vi "MAIN_GLD.vi"() -> ()   [LabVIEW 2019]
uses:
  <vilib>/platform/TimedLoop/XDataNode/XDataNode.xnode
  <vilib>/Platform/TimedLoop/XDataNode/nitl_modes.ctl
  <vilib>/Platform/TimedLoop/XDataNode/XDNodeRunTimeDep.lvlib
  <vilib>/Platform/TimedLoop/XDataNode/wakeup.ctl
  <vilib>/Platform/TimedLoop/XDataNode/timing_clust.ctl
  For fsr type def.ctl
  states typedef.ctl
  <vilib>/Analysis/NI_AALBase.lvlib
  <vilib>/Analysis/baseanly.llb/Mean (DBL).vi
  TESTtypedef UPDATED.ctl
  <extravilib>/ChannelInstances/Tag-bool.lvlib
  SineMinMax.ctl
  <vilib>/Instr/_visa.llb/VISA Configure Serial Port (Instr).vi
  weightTypedef.ctl
  groupID.ctl
  handInTest.ctl
  RampSlope.ctl
  RampHeight.ctl
panel:
  out "LF":dbl(graph)
  out "GF":dbl(graph)
  in  "Ramp's Height (N)":T1
  in  "Sine Min/Max (N)":T2=5.0
  out "Writing":bool
  in  "Stop Test":bool
  out "Grip Force [N]":cluster{"GF [N]":dbl}(graph)
  out "XY Graph":cluster{dbl[], dbl[]}[](graph)
  out "Test Time":dbl(graph)
  in  "Ramp's Width (s)":T3 caption="Test Type"
  in  "VISA":refnum<visa-resource-name>="COM1"
  out "Load Force [N]":cluster{"Dyna LF [N]":dbl}(graph)
  out "In Range?":bool
  in  "Wait time before beep (s)":dbl
  in  "Time b/w Beeps (s)":dbl=3.0
  in  "Stop":bool
  out "?":string
  in  "File Path":path=path "C:/Users/rsKite/Documents/Data_logs"
  out "Creating":bool
  in  "Create File":bool
  in  "Wrist Angle":enum16{"0", "30", "-30"}(ring)
  in  "Hand in Test":T4 caption="Test Type"
  in  "Trial":string caption="Participant Name (FirstLast)"
  in  "Patient ID":string caption="Participant Name (FirstLast)"
  in  "Group ID":T5
  in  "Weight":T6
  in  "Test Type":T7
  in  "Start Test":bool
  out "Calibrating":bool
  in  "Calibration":bool
  in  "Timer [ms]":u32=5000
  out "millisecond timer":u32
  out "dt":dbl
  out "millisecond timer 2":u32
  # "Status"
  # "Grip-Load Hand Assessment Device  Control Center"
  # "Control"
  # "Test Setup"
  # "File Control"
  # "Folder/File Information"
  # "STUFF THAT DOES NOT NEED TO BE DISPLAYED"
  # "Test Control"
  # "Force/Motion Trajectory Control"
  # "Test Time (s)"
  # "Grip Force"
  # "Load Force"
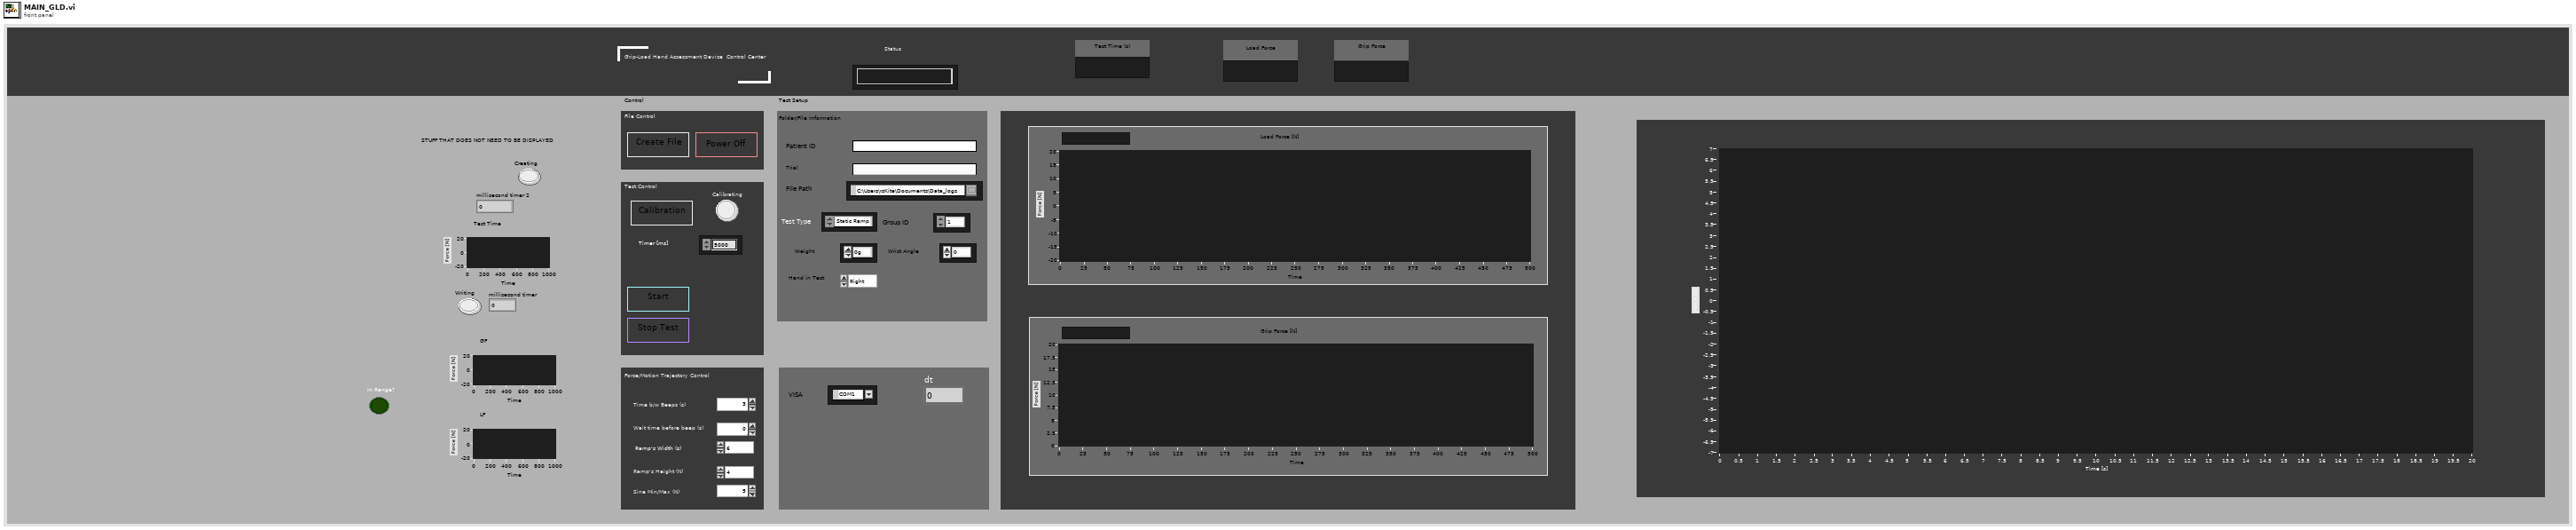
[diagram p1: front panel]
types:
  T1 = typedef "RampHeight.ctl" = enum16{"4", "5", "6"}
  T2 = typedef "SineMinMax.ctl" = dbl
  T3 = typedef "RampSlope.ctl" = enum16{"6", "5", "4"}
  T4 = typedef "handInTest.ctl" = enum16{"Right", "Left"}
  T5 = typedef "groupID.ctl" = enum16{"1", "2"}
  T6 = typedef "weightTypedef.ctl" = enum16{"0g", "300g", "600g", "900g"}
  T7 = typedef "TESTtypedef UPDATED.ctl" = enum16{"Static Ramp", "Static Sine", "Dynamic"}
  T8 = cluster{"String 2":string, dbl[], dbl[], dbl[], dbl[], dbl[], dbl[], dbl[], dbl[], "Test Type":T7, "Sine Min/Max (N) ":T2, "Ramp's Width":dbl, "Ramp's Height":dbl, dbl, dbl[]}
  T9 = typedef "states typedef.ctl" = enum16{"Init", "Create/Replace", "Calibration", "Ready?", "Testing", "Write Data", "Restart"}
  T10 = typedef "For fsr type def.ctl" = enum16{"Create/Replace File", "Waiting Room", "Collect Data", "Write Data", "Close File", "Reinit"}
  T11 = typedef "XDNodeRunTimeDep.lvlib/timing_clust.ctl" = cluster{"Expected End [f-1]":u64, "Actual End [f-1]":u64, "Finished Late? [f-1]":bool, "Expected End [i-1]":u64, "Actual End [i-1]":u64, "Finished Late? [i-1]":bool, "Expected Start [i]":u64, "Actual Start [i]":u64, "Expected Start [f]":u64, "Actual Start [f]":u64, "Source Name":string, "Structure Name":string, "Period":i64, "Deadline":i64, "Offset":i64, "Start":i64, "Priority":i32, "Timeout":i32, "Mode":T12, "Wakeup Reason":T13, "Error":errorcluster, "Source Type":string, "Secondary Source Type":string, "Global End Time":u64, "Global Start Time":u64, "Frame Duration":u64, "Iteration Duration":u64, "Assigned CPU":i32, "I/O Scan Engine Mode":u32}
  T12 = typedef "XDNodeRunTimeDep.lvlib/nitl_modes.ctl" = enum32{"No Change", "Process missed periods, maintain original phase", "Discard missed periods, maintain original phase", "Process missed periods, ignore original phase", "Discard missed periods, ignore original phase"}
  T13 = typedef "XDNodeRunTimeDep.lvlib/wakeup.ctl" = enum32{"Normal", "Aborted", "Asynchronous wakeup", "Timing source error", "Timed loop error", "Timeout"}
  T14 = cluster{"Foldername and filename string":string, dbl[], dbl[], dbl[], dbl[], "output array":dbl[], "output array":dbl[], "output array":dbl[], "output array":dbl[], "Test Type":T7, "Sine Min/Max (N) ":T2, "Ramp's Width":dbl, "Ramp's Height":dbl, dbl, "output array":dbl[]}
  T15 = cluster{"String 2":string, dbl[], dbl[], dbl[], dbl[], "array":dbl[], dbl[], dbl[], "output array":dbl[], "Test Type":T7, "Sine Min/Max (N) ":T2, "Ramp's Width":dbl, "Ramp's Height":dbl, dbl, dbl[]}
  T16 = cluster{"String 2":string, dbl[], dbl[], dbl[], dbl[], "array":dbl[], "output array":dbl[], "output array":dbl[], dbl[], "Test Type":T7, "Sine Min/Max (N) ":T2, "Ramp's Width":dbl, "Ramp's Height":dbl, dbl, "output array":dbl[]}
  T17 = typedef "Tag-bool.lvlib/))Channel.ctl" = refnum<queue>
  T18 = cluster{"refnum out":refnum<file>, "error out":errorcluster}
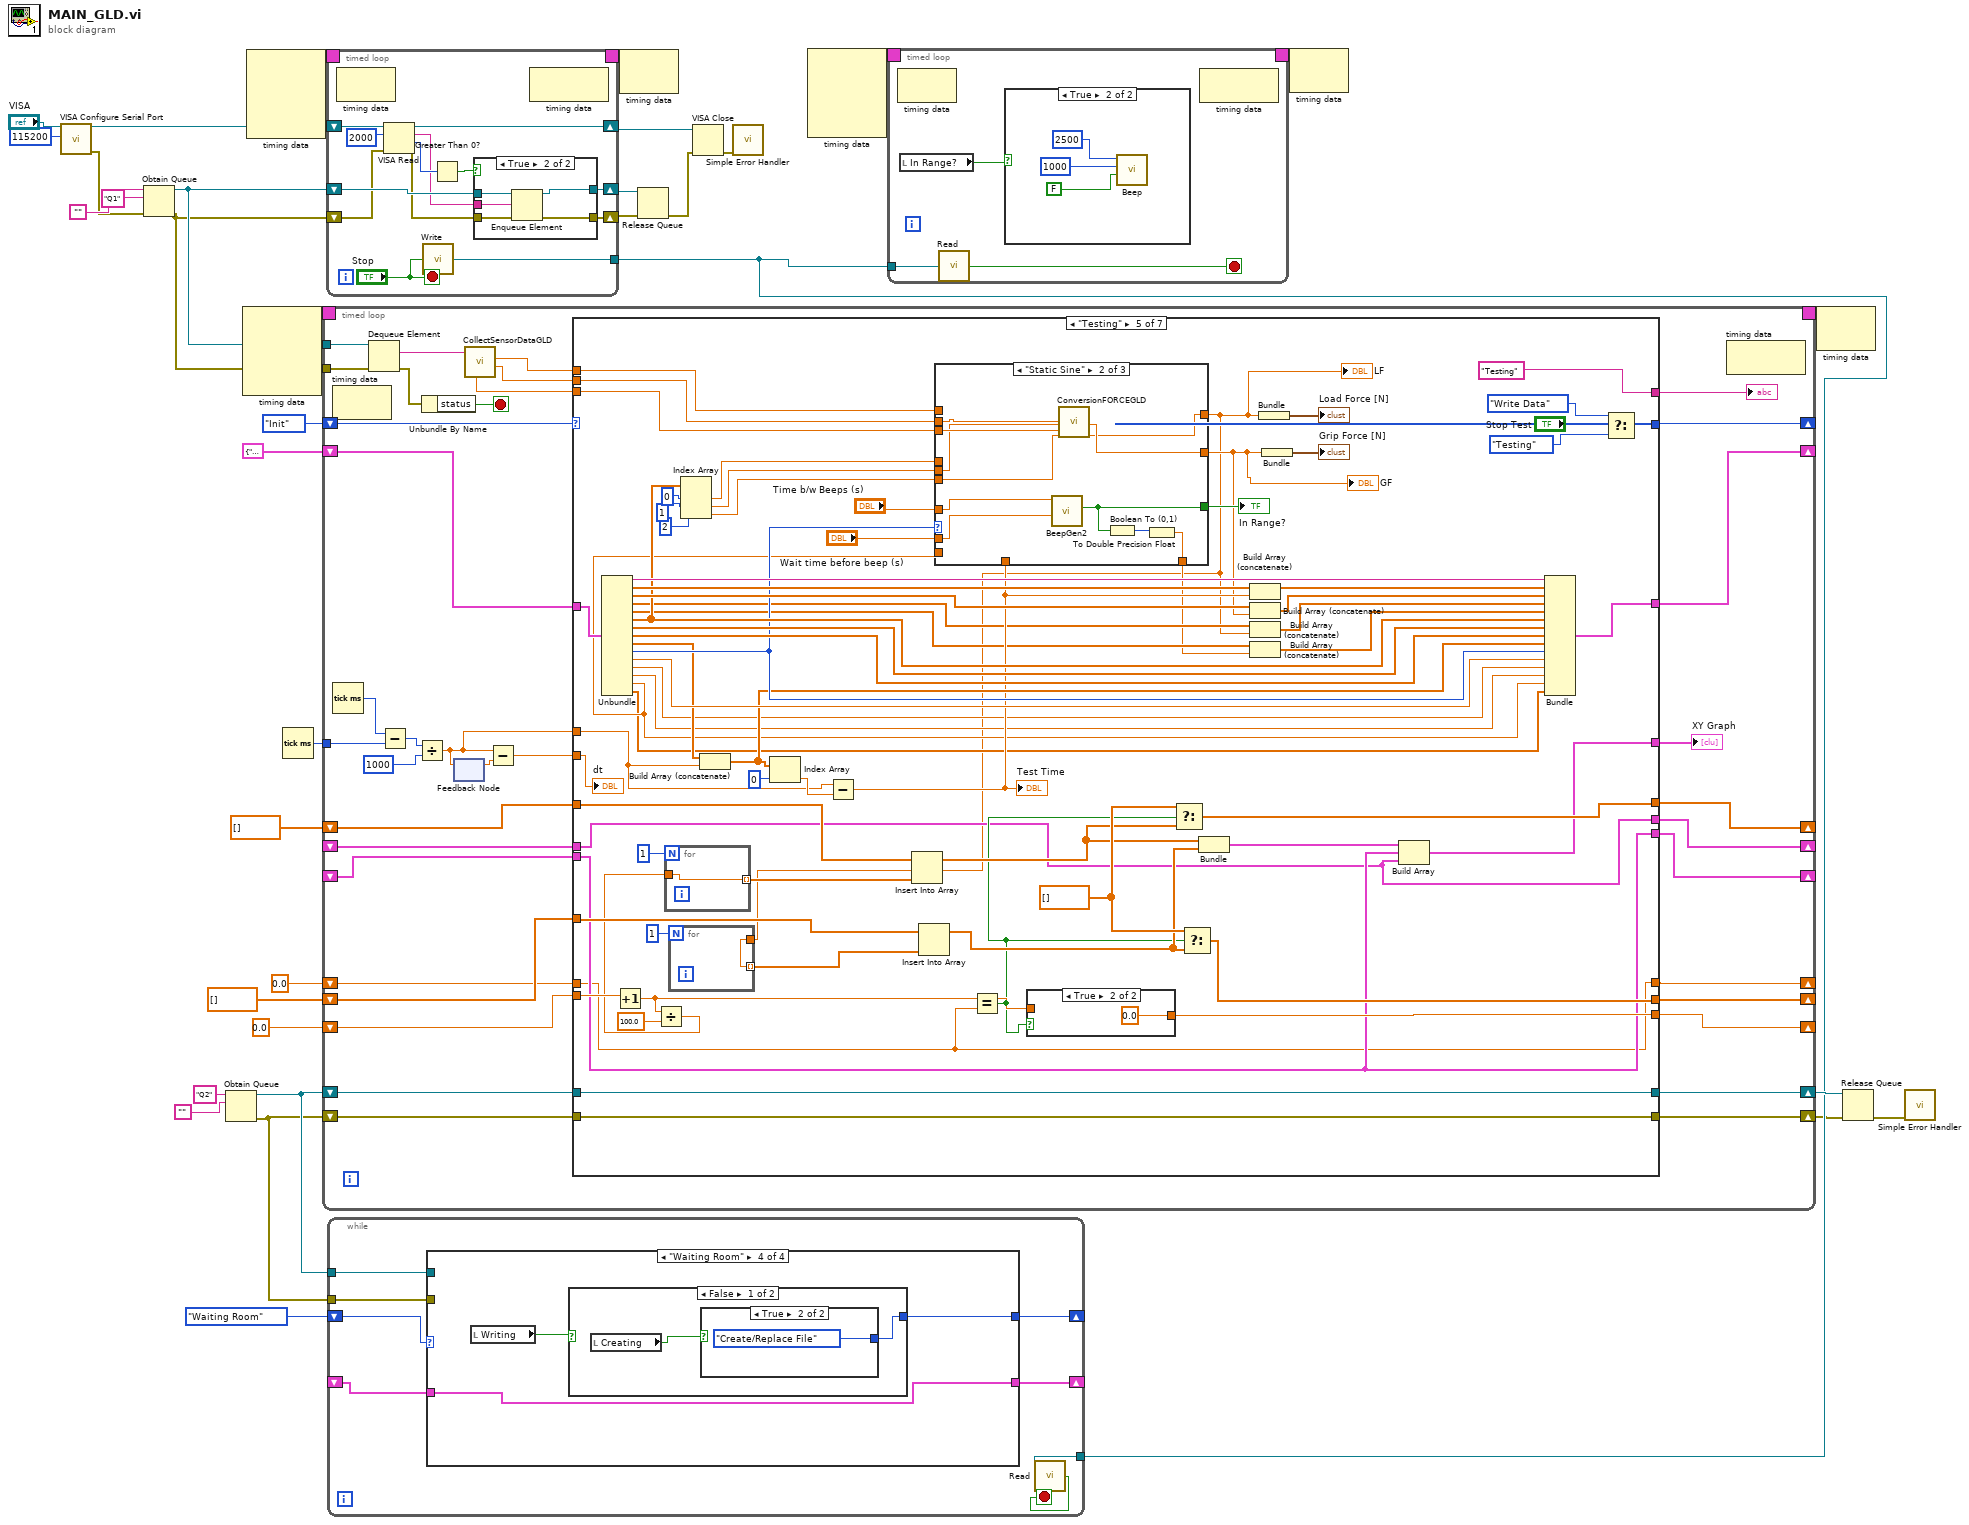
[diagram p0: block diagram]
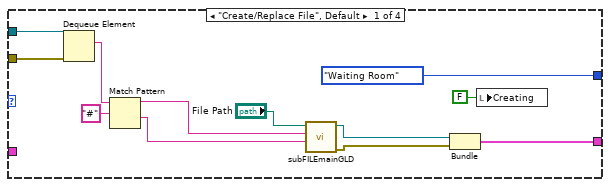
[diagram p3: hidden frame]
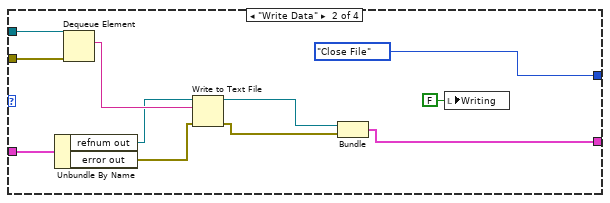
[diagram p4: hidden frame]
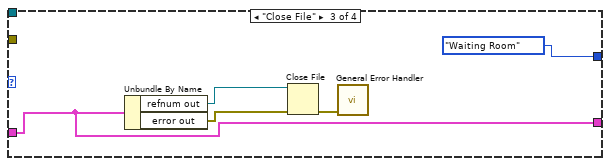
[diagram p5: hidden frame]
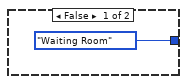
[diagram p6: hidden frame]
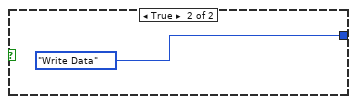
[diagram p7: hidden frame]
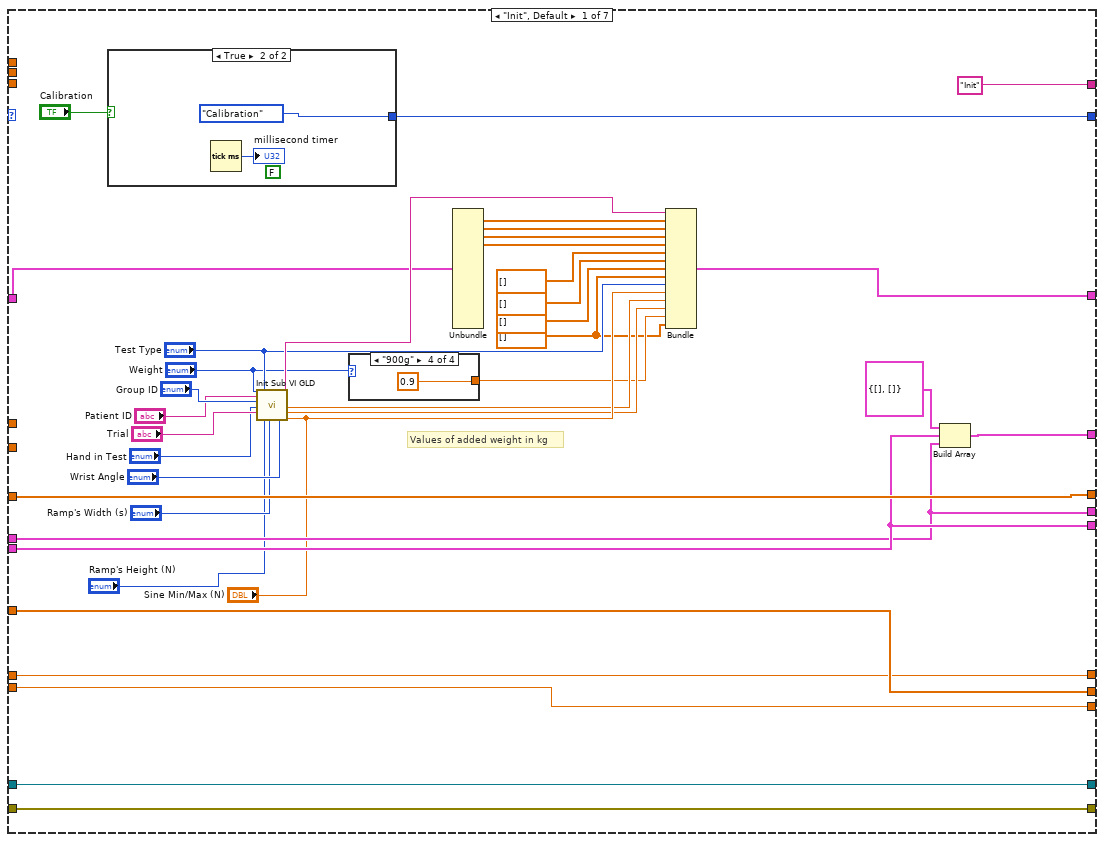
[diagram p8: hidden frame]
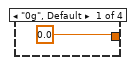
[diagram p9: hidden frame]
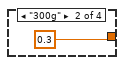
[diagram p10: hidden frame]
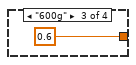
[diagram p11: hidden frame]
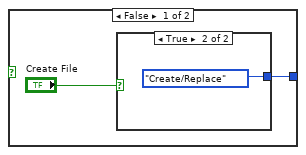
[diagram p12: hidden frame]
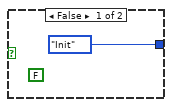
[diagram p13: hidden frame]
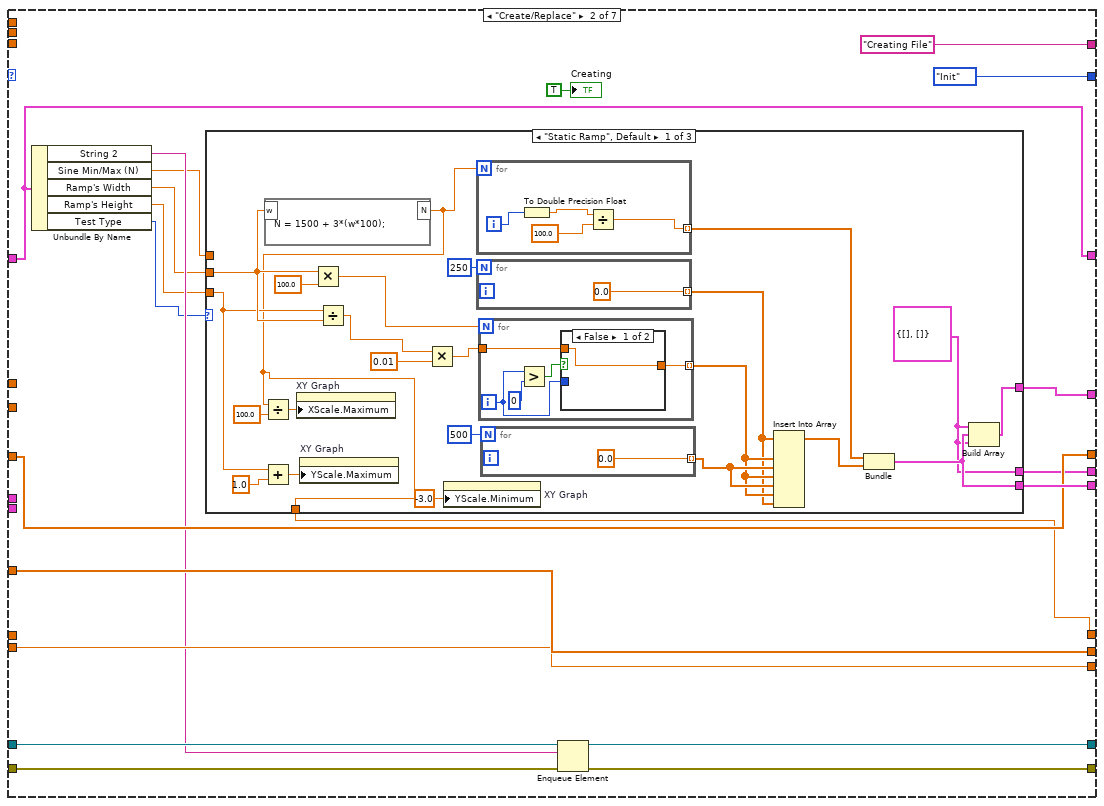
[diagram p14: hidden frame]
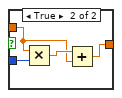
[diagram p15: hidden frame]
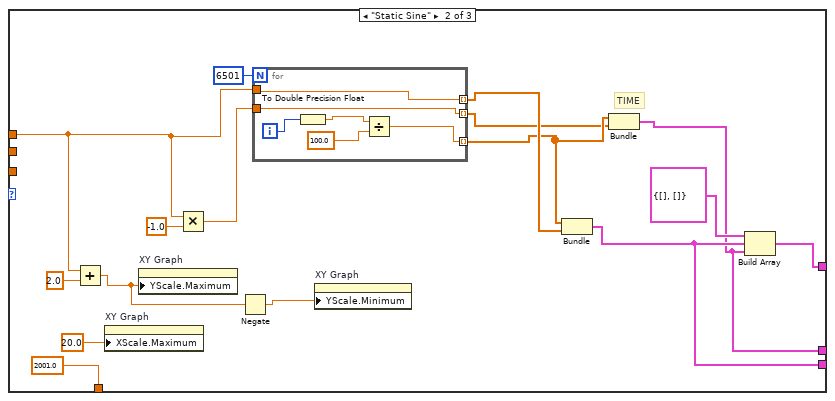
[diagram p16: hidden frame]
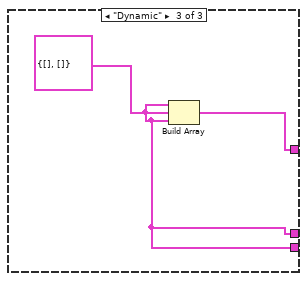
[diagram p17: hidden frame]
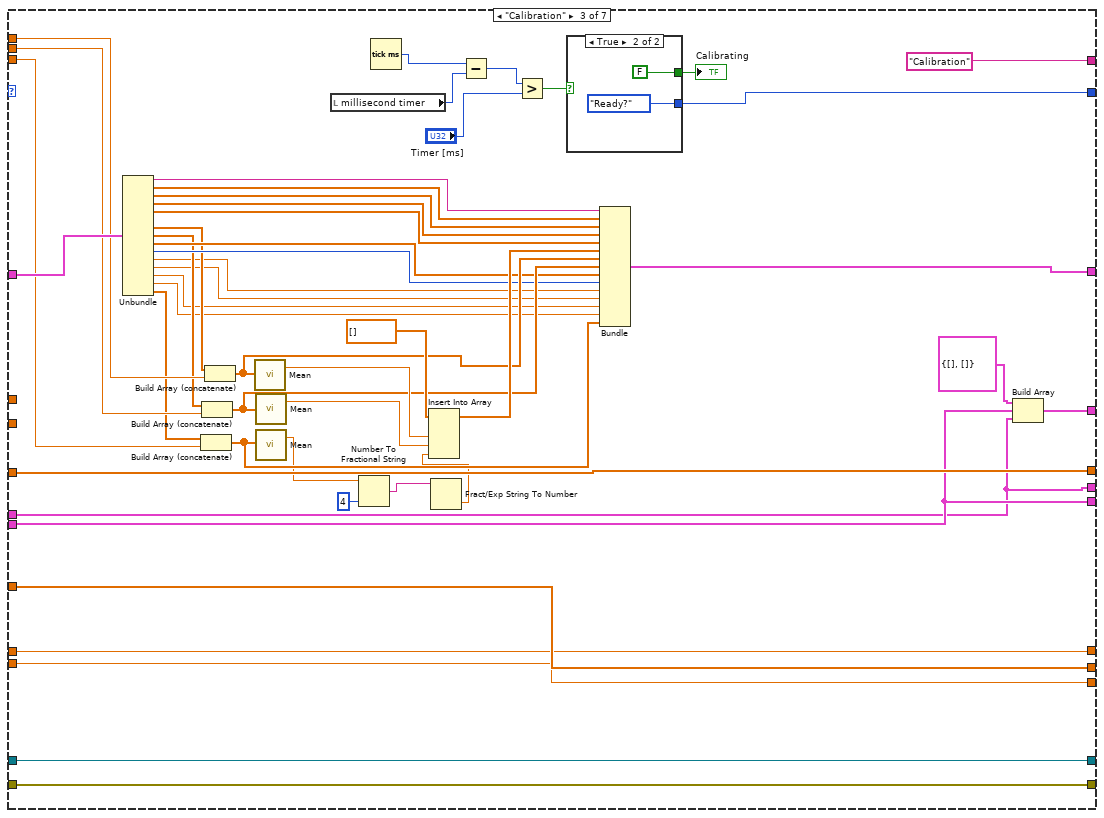
[diagram p18: hidden frame]
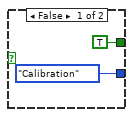
[diagram p19: hidden frame]
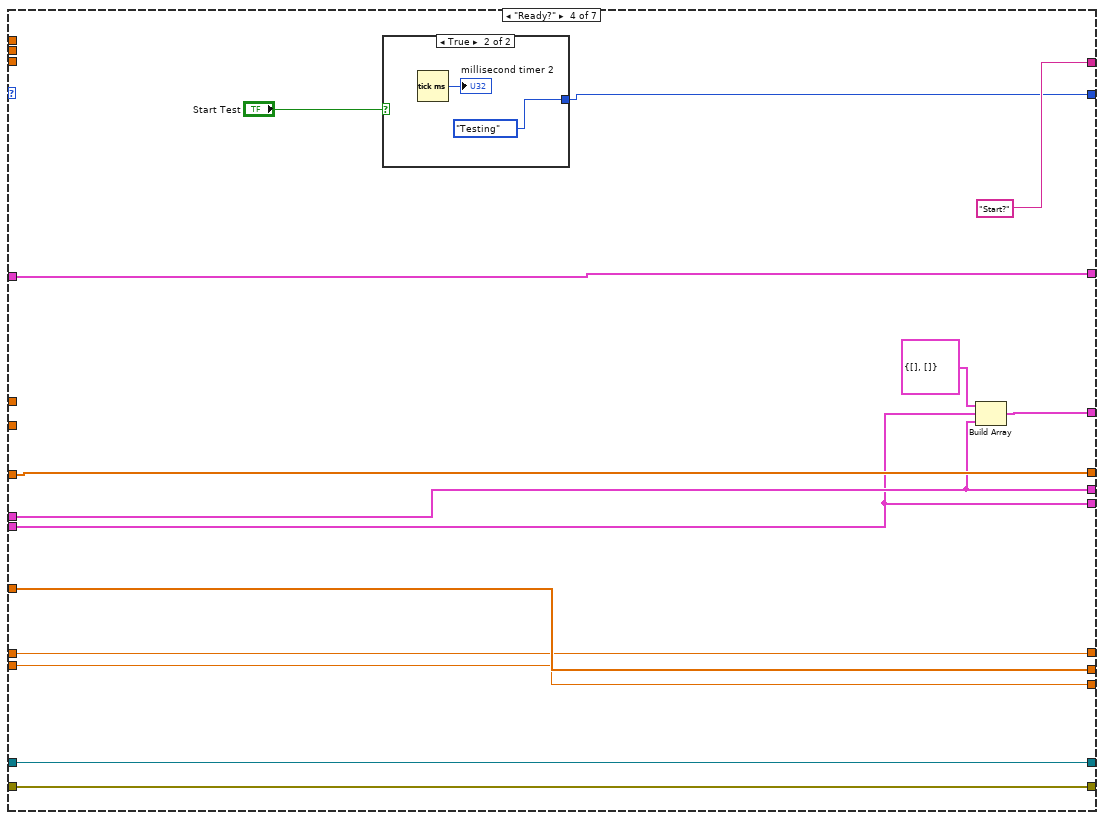
[diagram p20: hidden frame]
diagram:
  n1 = call-poly "VISA Configure Serial Port"("VISA resource name"="VISA", "baud rate (9600)"=u32 115200) -> ("VISA resource name out"=w31:refnum<visa-resource-name>, "error out"=w26:errorcluster)  [unwired: 12 in]
  n2 = Obtain Queue(name (unnamed)="Q1", element data type="", error in (no error)=w26) -> (queue out=w33:refnum<queue>, error out=w32:errorcluster)  [unwired: 2 in, 1 out]
  n3 = Obtain Queue(name (unnamed)="Q2", element data type="") -> (queue out=w17:refnum<queue>, error out=w16:errorcluster)  [unwired: 3 in, 1 out]
  n4 = node-c288() -> (w21:T11)  [unwired: 4 in]
  n5 = node-c288() -> (w23:T11)  [unwired: 4 in]
  n6 = Tick Count (ms)() -> (millisecond timer value=w24:u32)
  n7 = timed-loop {
    tunnel: w33 -> [w72]
    tunnel: w32 -> [w71]
    tunnel: w24 -> [w68]
    timing: w21 -> [_]
    timing-out: [_] -> w20
    shift-right: [w60] -> _
    shift-left: states_typedef."Init" -> [w59]
    shift-right: [w62] -> w15
    shift-left: w17 -> [w64]
    shift-right: [w61] -> w2
    shift-left: w16 -> [w63]
    shift-right: [w56] -> _
    shift-left: T8 {"String 2"="", [], [], [], [], [], [], [], [], "Test Type"=enum."Dynamic", "Sine Min/Max (N) "=3000.0, "Ramp's Width"=0.0, "Ramp's Height"=0.0, 0.0, []} -> [w57]
    shift-right: [w53] -> _
    shift-left: _ -> [w52]
    shift-right: [w45] -> _
    shift-left: dbl[] [] ("t") -> [w46]
    shift-right: [w44] -> _
    shift-left: dbl[] [] ("t") -> [w43]
    shift-right: [w40] -> _
    shift-left: 0.0 -> [w41]
    shift-right: [w39] -> _
    shift-left: _ -> [w38]
    shift-right: [w37] -> _
    shift-left: 0.0 ("Y Scale.Range:Maximum") -> [w36]
    stop <- w55 stop-if-true
    n8 = node-c288() -> ()  [unwired: 1 in, 1 out]
    n9 = Tick Count (ms)() -> (millisecond timer value=w69:u32)
    n10 = Dequeue Element(queue=w72, error in (no error)=w71) -> (element=w58:string, error out=w70:errorcluster)  [unwired: 1 in, 2 out]
    n11 = Subtract(x=w69, y=w68) -> (x-y=w66:u32)
    n12 = Divide(x=w66, y=1000) -> (x/y=w51:dbl)
    n13 = Unbundle By Name(w70) -> ("status"=w55:bool)
    n14 = feedback-in #1(w51) -> ()
    n15 = feedback #1() -> (w65:dbl)  [unwired: 1 in]
    n16 = call "CollectSensorDataGLD.vi"("data (can be any type)"=w58) -> ("grams (GF)"=w47:dbl, "Accel (Dyna LF)"=w48:dbl, "Volt (Static LF)"=w49:dbl)  [unwired: 8 in]
    n17 = Subtract(x=w51, y=w65) -> (x-y=w50:dbl)
    n18 = case shown="\"Testing\"" w59 {
      tunnel: [w109 states_typedef."Init" w241 w263 w313 states_typedef."Restart" states_typedef."Init"] -> w60
      tunnel: w64 -> [w107 w139 w240 w267 w344 w409 w426]
      tunnel: w63 -> [w106 w121 w239 w266 w343 w408 w425]
      tunnel: [w107 w138 w240 w267 w344 w407 w426] -> w62
      tunnel: [w106 w137 w239 w266 w343 w406 w425] -> w61
      tunnel: w57 -> [w90 w127 w238 w265 w340 w404 _]
      tunnel: [w95 w127 w231 w265 w335 w404 T8 {"String 2"="", [], [], [], [], [], [], [], [], "Test Type"=enum."Dynamic", "Sine Min/Max (N) "=3000.0, "Ramp's Width"=0.0, "Ramp's Height"=0.0, 0.0, []}] -> w56
      tunnel: ["Init" "Creating File" "Calibration" "Start?" "Testing" "Logging" "Restarting"] -> w54
      tunnel: [w86 w133 w217 w256 w290 w396 w420] -> w53
      tunnel: w52 -> [w86 _ w217 w256 w290 w396 w420]
      tunnel: w51 -> [_ _ _ _ w331 _ _]
      tunnel: w48 -> [_ _ w229 _ w330 _ _]
      tunnel: w50 -> [_ _ _ _ w329 _ _]
      tunnel: w49 -> [_ _ w210 _ w325 _ _]
      tunnel: w47 -> [_ _ w211 _ w326 _ _]
      tunnel: w46 -> [w88 w132 w221 w261 w307 w399 _]
      tunnel: [w88 w132 w221 w261 w309 w399 dbl[] [] ("t")] -> w45
      tunnel: [w87 w131 w220 w262 w308 w398 dbl[] [] ("t")] -> w44
      tunnel: w43 -> [w87 w131 w220 w262 w304 w398 _]
      tunnel: [w85 w130 w213 w260 w298 w397 w419] -> w42
      tunnel: w41 -> [w84 w129 w219 w259 w297 w395 _]
      tunnel: [w84 w129 w219 w259 w296 w395 0.0] -> w40
      tunnel: [w81 w128 w216 w257 w289 w393 w416] -> w39
      tunnel: w38 -> [w81 _ w216 w257 w289 w393 w416]
      tunnel: [w73 w120 w203 w255 w274 w383 0.0 ("Y Scale.Range:Maximum")] -> w37
      tunnel: w36 -> [w73 _ w203 w255 w274 w383 _]
      frame "Init", Default {
        w74 = dbl[] [] ("output array")
        # "Values of added weight in kg"
        n19 = case shown="True" "Calibration" {
          tunnel: [w115 states_typedef."Calibration"] -> w109
          frame False {
            n20 = case shown="True" "Create File" {
              tunnel: [states_typedef."Init" states_typedef."Create/Replace"] -> w115
              frame False {
                (unwired) FALSE
              }
              frame True {
              }
            }
          }
          frame True {
            (unwired) FALSE
            n21 = Tick Count (ms)() -> (millisecond timer value=→"millisecond timer":u32)
          }
        }
        n22 = call "Init Sub VI GLD.vi"("Weight"="Weight", "Patient ID"="Patient ID", "Group ID"="Group ID", "Hand in Test"="Hand in Test", "Trial"="Trial", "Test Type"="Test Type", "Ramp's Height (N)"="Ramp's Height (N)", "Ramp's Width (s)"="Ramp's Width (s)", "Wrist Angle"="Wrist Angle", "Sine Min/Max"="Sine Min/Max (N)") -> ("Foldername and filename string"=w94:string, "Ramp's Width"=w78:dbl, "Ramp's Height"=w77:dbl)  [unwired: 6 in, 1 out]
        n23 = case shown="\"900g\"" "Weight" {
          tunnel: [0.0 0.3 0.6 0.9] -> w75
          frame "0g", Default {
          }
          frame "300g" {
          }
          frame "600g" {
          }
          frame "900g" {
          }
        }
        n24 = Unbundle(w90) -> (w100:dbl[], w99:dbl[], w98:dbl[], w97:dbl[])  [unwired: 11 out]
        n25 = Bundle("Foldername and filename string"=w94, w100, w99, w98, w97, "output array"=dbl[] [], "output array"=dbl[] [], "output array"=dbl[] [], "output array"=w74, "Test Type"="Test Type", "Sine Min/Max (N)"="Sine Min/Max (N)", "Ramp's Width"=w78, "Ramp's Height"=w77, w75, "output array"=w74) -> (w95:T14)  [unwired: 1 in]
        n26 = Build Array(cluster{dbl[], dbl[]} {[], []} ("element"), w86, w81) -> (w85:cluster{dbl[], T2[]}[])
      }
      frame "Create/Replace" {
        n27 = Unbundle By Name(w127) -> ("String 2"=w126:string, "Sine Min/Max (N)"=w124:T2, "Ramp's Width"=w123:dbl, "Ramp's Height"=w122:dbl, "Test Type"=w125:T7)
        n28 = case shown="\"Static Ramp\", Default" w125 {
          tunnel: [w161 w193 w201] -> w133
          tunnel: w123 -> [w147 _ _]
          tunnel: [w159 w194 w202] -> w130
          tunnel: w124 -> [_ w183 _]
          tunnel: [w158 w187 w201] -> w128
          tunnel: w122 -> [w145 _ _]
          tunnel: [w141 2001.0 ("Y Scale.Range:Maximum") _] -> w120
          frame "Static Ramp", Default {
            w158 = cluster{dbl[], dbl[]} {[], []} ("element")
            n29 = Add(x=w145, y=1.0) -> (x+y=w143:dbl)
            n30 = formula code="N = 1500 + 3*(w*100);"("w"=w147) -> ("N"=w141:dbl)
            n31 = Divide(x=w141, y=100.0) -> (x/y=w142:dbl)
            n32 = property on="XY Graph" class="XYGraph (strict)"("XScale.Maximum"=w142) -> ()  [unwired: 2 in, 2 out]
            n33 = property on="XY Graph" class="XYGraph (strict)"("YScale.Maximum"=w143) -> ()  [unwired: 2 in, 2 out]
            n34 = Multiply(x=w147, y=100.0) -> (x*y=w155:dbl)
            n35 = Divide(x=w145, y=w147) -> (x/y=w153:dbl)
            n36 = Multiply(x=w153, y=0.01) -> (x*y=w152:dbl)
            n37 = property on="XY Graph" class="XYGraph (strict)"("YScale.Minimum"=-3.0 ("Y Scale.Range:Minimum")) -> ()  [unwired: 2 in, 2 out]
            n38 = for {
              N: w141 -> [_]
              tunnel: [w175] -> w157 mode=indexing
              i -> [w178]
              n39 = To Double Precision Float(number=w178) -> (double precision float=w176:dbl)
              n40 = Divide(x=w176, y=100.0) -> (x/y=w175:dbl)
            }
            n41 = for {
              N: 250 -> [_]
              tunnel: [0.0] -> w148 mode=indexing
            }
            n42 = for {
              N: w155 -> [_]
              tunnel: w152 -> [w166]
              tunnel: [w165] -> w149 mode=indexing
              i -> [w164]
              n43 = Greater?(x=w164, y=0) -> (0:w167:bool)
              n44 = case shown="False" w167 {
                tunnel: w166 -> [w169 w171]
                tunnel: [w169 w170] -> w165
                tunnel: w164 -> [_ w173]
                frame False {
                }
                frame True {
                  n45 = Multiply(x=w171, y=w173) -> (x*y=w172:dbl)
                  n46 = Add(x=w172, y=w171) -> (x+y=w170:dbl)
                }
              }
            }
            n47 = for {
              N: 500 -> [_]
              tunnel: [0.0] -> w150 mode=indexing
            }
            n48 = Insert Into Array(array=w148, new element #1=w149, new element #2=w150, new element #3=w149, new element #4=w150, new element #5=w149, new element #6=w148) -> (w162:dbl[])  [unwired: 1 in]
            n49 = Bundle(w157, w162) -> (w161:cluster{dbl[], dbl[]})  [unwired: 1 in]
            n50 = Build Array(w158, w161, w158) -> (w159:cluster{dbl[], dbl[]}[])
          }
          frame "Static Sine" {
            # "TIME"
            n51 = Add(x=w183, y=2.0) -> (x+y=w181:T2)
            n52 = property on="XY Graph" class="XYGraph (strict)"("XScale.Maximum"=20.0 ("Y Scale.Range:Maximum")) -> ()  [unwired: 2 in, 2 out]
            n53 = property on="XY Graph" class="XYGraph (strict)"("YScale.Maximum"=w181) -> ()  [unwired: 2 in, 2 out]
            n54 = Multiply(x=w183, y=-1.0) -> (x*y=w185:T2)
            n55 = Negate(x=w181) -> (-x=w180:T2)
            n56 = for {
              N: 6501 -> [_]
              tunnel: [w196] -> w192 mode=indexing
              tunnel: [w197] -> w191 mode=indexing
              tunnel: w183 -> [w196]
              tunnel: w185 -> [w195]
              tunnel: [w195] -> w186 mode=indexing
              i -> [w200]
              n57 = To Double Precision Float(number=w200) -> (double precision float=w198:dbl)
              n58 = Divide(x=w198, y=100.0) -> (x/y=w197:dbl)
            }
            n59 = property on="XY Graph" class="XYGraph (strict)"("YScale.Minimum"=w180) -> ()  [unwired: 2 in, 2 out]
            n60 = Bundle(w191, w192) -> (w193:cluster{dbl[], T2[]})  [unwired: 1 in]
            n61 = Bundle(w191, w186) -> (w187:cluster{dbl[], T2[]})  [unwired: 1 in]
            n62 = Build Array(cluster{dbl[], T2[]} {[], []} ("element"), w193, w187) -> (w194:cluster{dbl[], T2[]}[])
          }
          frame "Dynamic" {
            w201 = cluster{dbl[], dbl[]} {[], []} ("element")
            n63 = Build Array(w201, w201, w201) -> (w202:cluster{dbl[], dbl[]}[])
          }
        }
        n64 = Enqueue Element(queue=w139, element=w126, error in (no error)=w121) -> (queue out=w138:refnum<queue>, error out=w137:errorcluster)  [unwired: 1 in, 1 out]
        "Creating" <- TRUE ("Creating")
      }
      frame "Calibration" {
        n65 = Unbundle(w238) -> ("String 2"=w237:string, w236:dbl[], w235:dbl[], w234:dbl[], w233:dbl[], "output array"=w224:dbl[], "output array"=w223:dbl[], "output array"=w226:dbl[], "Test Type"=w225:T7, "Sine Min/Max (N)"=w222:T2, "Ramp's Width"=w215:dbl, "Ramp's Height"=w214:dbl, w212:dbl, "output array"=w209:dbl[])  [unwired: 1 out]
        n66 = Build Array (concatenate)(w209, w210) -> (w208:dbl[])
        n67 = Build Array (concatenate)(w223, w211) -> (w227:dbl[])
        n68 = Build Array (concatenate)(w224, w229) -> (w228:dbl[])
        n69 = call-poly <vilib>:"Mean.vi"("X"=w228) -> ("mean"=w249:dbl)  [unwired: 1 out]
        n70 = call-poly <vilib>:"Mean.vi"("X"=w227) -> ("mean"=w248:dbl)  [unwired: 1 out]
        n71 = call-poly <vilib>:"Mean.vi"("X"=w208) -> ("mean"=w206:dbl)  [unwired: 1 out]
        n72 = local read "millisecond timer"() -> (w246:u32)
        n73 = Number To Fractional String(number=w206, precision (6)=i16 4) -> (F-format string=w205:string)  [unwired: 2 in]
        n74 = Tick Count (ms)() -> (millisecond timer value=w247:u32)
        n75 = Fract/Exp String To Number(string=w205) -> (number=w204:dbl)  [unwired: 3 in, 1 out]
        n76 = Insert Into Array(array=dbl[] [], new element #1=w249, new element #2=w248, new element #3=w204) -> (w232:dbl[])  [unwired: 1 in]
        n77 = Subtract(x=w247, y=w246) -> (x-y=w244:u32)
        n78 = Greater?(x=w244, y="Timer [ms]") -> (0:w243:bool)
        n79 = case shown="True" w243 {
          tunnel: [TRUE FALSE] -> w242
          tunnel: [states_typedef."Calibration" states_typedef."Ready?"] -> w241
          frame False {
          }
          frame True {
          }
        }
        "Calibrating" <- w242
        n80 = Bundle("String 2"=w237, w236, w235, w234, w233, "array"=w232, w228, w227, "output array"=w226, "Test Type"=w225, "Sine Min/Max (N)"=w222, "Ramp's Width"=w215, "Ramp's Height"=w214, w212, w208) -> (w231:T15)  [unwired: 1 in]
        n81 = Build Array(cluster{dbl[], dbl[]} {[], []} ("element"), w217, w216) -> (w213:cluster{dbl[], T2[]}[])
      }
      frame "Ready?" {
        n82 = case shown="True" "Start Test" {
          tunnel: [states_typedef."Ready?" states_typedef."Testing"] -> w263
          frame False {
          }
          frame True {
            n83 = Tick Count (ms)() -> (millisecond timer value=→"millisecond timer 2":u32)
          }
        }
        n84 = Build Array(cluster{dbl[], dbl[]} {[], []} ("element"), w256, w257) -> (w260:cluster{dbl[], T2[]}[])
      }
      frame "Testing" {
        w310 = dbl[] [] ("t")
        n85 = Unbundle(w340) -> ("String 2"=w339:string, w338:dbl[], w337:dbl[], w281:dbl[], w279:dbl[], "array"=w336:dbl[], "output array"=w327:dbl[], "output array"=w323:dbl[], "output array"=w320:dbl[], "Test Type"=w322:T7, "Sine Min/Max (N)"=w321:T2, "Ramp's Width"=w285:dbl, "Ramp's Height"=w284:dbl, w276:dbl, "output array"=w275:dbl[])
        n86 = Increment(x=w297) -> (x+1=w295:dbl)
        n87 = Divide(x=w295, y=100.0) -> (x/y=w293:dbl)
        n88 = for {
          N: 1 -> [_]
          tunnel: w293 -> [w345]
          tunnel: [w345] -> w292 mode=indexing
        }
        n89 = Index Array(array=w336, index #1=0 ("index"), index #2=1 ("index"), index #3=2 ("index")) -> (element #1=w328:dbl, element #2=w324:dbl, element #3=w317:dbl)
        n90 = Build Array (concatenate)(w320, w331) -> (w319:dbl[])
        n91 = Index Array(array=w319, index=0) -> (element=w332:dbl)
        n92 = Subtract(x=w331, y=w332) -> (x-y=w301:dbl)
        "Test Time" <- w301
        n93 = Insert Into Array(array=w307, new element=w292) -> (w299:dbl[])  [unwired: 1 in]
        n94 = case shown="\"Static Sine\"" w322 {
          tunnel: w330 -> [w358 _ w382]
          tunnel: [w350 w364 w380] -> w272
          tunnel: w328 -> [w357 _ w381]
          tunnel: w326 -> [w353 w359 w379]
          tunnel: w325 -> [w355 w369 _]
          tunnel: w324 -> [w352 w360 w378]
          tunnel: w317 -> [w356 w368 _]
          tunnel: w301 -> [_ _ w377]
          tunnel: [FALSE ("In Range?") w363 w372] -> w288
          tunnel: "Time b/w Beeps (s)" -> [_ w367 w376]
          tunnel: "Wait time before beep (s)" -> [_ w366 w375]
          tunnel: [w351 w365 w374] -> w273
          tunnel: [0.0 w361 w371] -> w277
          tunnel: w276 -> [_ _ w370]
          frame "Static Ramp", Default {
            n95 = call "ConversionFORCEGLD.vi"("Accel (Dyna LF)"=w358, "Accel (Dyna LF) Offset"=w357, "grams (Omega GF)"=w353, "grams (Omega GF) Offset"=w352, "Futek  (Static LF)"=w355, "Futek  (Static LF) Offset"=w356) -> ("GF [N]"=w351:dbl, "Static LF [N]"=w350:dbl)  [unwired: 11 in, 1 out]
          }
          frame "Static Sine" {
            n96 = call "BeepGen2.vi"("Wait time before beep (s)"=w366, "Time b/w Beeps (s)"=w367) -> ("In Range?"=w363:bool)  [unwired: 7 in, 2 out]
            n97 = call "ConversionFORCEGLD.vi"("grams (Omega GF)"=w359, "grams (Omega GF) Offset"=w360, "Futek  (Static LF)"=w369, "Futek  (Static LF) Offset"=w368) -> ("GF [N]"=w365:dbl, "Static LF [N]"=w364:dbl)  [unwired: 13 in, 1 out]
            n98 = Boolean To (0,1)(Boolean=w363) -> (0, 1=w362:i16)
            n99 = To Double Precision Float(number=w362) -> (double precision float=w361:dbl)
          }
          frame "Dynamic" {
            n100 = call "ConversionFORCEGLD.vi"("Accel (Dyna LF)"=w382, "Accel (Dyna LF) Offset"=w381, "grams (Omega GF)"=w379, "grams (Omega GF) Offset"=w378, "Weight added (kg)"=w370) -> ("Dyna LF [N]"=w380:dbl, "GF [N]"=w374:dbl)  [unwired: 12 in, 1 out]
            n101 = call "BeepGen.vi"("Numeric in"=w377, "Wait time before beep"=w375, "Time b/w Beeps (ms)"=w376) -> ("In Range?"=w372:bool)  [unwired: 7 in, 1 out]
            n102 = Boolean To (0,1)(Boolean=w372) -> (0, 1=w373:i16)
            n103 = To Double Precision Float(number=w373) -> (double precision float=w371:dbl)
          }
        }
        "In Range?" <- w288
        "GF" <- w273
        "LF" <- w272
        n104 = for {
          N: 1 -> [_]
          tunnel: w272 -> [w348]
          tunnel: [w348] -> w305 mode=indexing
        }
        n105 = Insert Into Array(array=w304, new element=w305) -> (w303:dbl[])  [unwired: 1 in]
        n106 = Equal?(x=w295, y=w274) -> (x = y?=w291:bool)
        n107 = case shown="True" w291 {
          tunnel: w295 -> [w346 _]
          tunnel: [w346 0.0] -> w296
          frame False {
          }
          frame True {
          }
        }
        n108 = Select(t=w310, s=w291, f=w299) -> (s? t:f=w309:dbl[])
        n109 = Select(t=w310, s=w291, f=w303) -> (s? t:f=w308:dbl[])
        n110 = Bundle("t"=w299, "t"=w303) -> (w300:cluster{"t":dbl[], "t":dbl[]})  [unwired: 1 in]
        n111 = Build Array (concatenate)(w338, w301) -> (w312:dbl[])
        n112 = Build Array (concatenate)(w337, w273) -> (w302:dbl[])
        n113 = Build Array (concatenate)(w281, w272) -> (w280:dbl[])
        n114 = Build Array (concatenate)(w279, w277) -> (w278:dbl[])
        n115 = Bundle("Dyna LF [N]"=w272) -> (→"Load Force [N]":cluster{"Dyna LF [N]":dbl})  [unwired: 1 in]
        n116 = Bundle("GF [N]"=w273) -> (→"Grip Force [N]":cluster{"GF [N]":dbl})  [unwired: 1 in]
        n117 = Build Array(w300, w290, w289) -> (w298:cluster{"t":dbl[], "t":T2[]}[])
        n118 = Bundle("String 2"=w339, w312, w302, w280, w278, "array"=w336, "output array"=w327, "output array"=w323, w319, "Test Type"=w322, "Sine Min/Max (N)"=w321, "Ramp's Width"=w285, "Ramp's Height"=w284, w276, "output array"=w275) -> (w335:T16)  [unwired: 1 in]
        n119 = Select(t=states_typedef."Write Data", s="Stop Test", f=states_typedef."Testing") -> (s? t:f=w313:T9)
        "dt" <- w329
      }
      frame "Write Data" {
        w389 = "\t"
        n120 = Unbundle(w404) -> (w403:dbl[], w402:dbl[], w385:dbl[], w384:dbl[])  [unwired: 11 out]
        n121 = Build Array(w403, w402, w385, w384) -> (w413:dbl[][])
        n122 = Transpose Matrix(1:w413) -> (0:w412:dbl[][])
        n123 = Array To Spreadsheet String(array=w412, 3:"%5.3f" ("format string")) -> (spreadsheet string=w386:string)  [unwired: 1 in]
        n124 = Concatenate Strings("time (s)" ("string"), w389, "Grip Force [N]" ("string"), w389, "Load Force [N]" ("string"), w389, "Flag Occurence" ("string"), "\r\n", w386) -> (w410:string)
        n125 = Enqueue Element(queue=w409, element=w410, error in (no error)=w408) -> (queue out=w407:refnum<queue>, error out=w406:errorcluster)  [unwired: 1 in, 1 out]
        n126 = Build Array(cluster{dbl[], dbl[]} {[], []} ("element"), w396, w393) -> (w397:cluster{dbl[], T2[]}[])
        "Writing" <- TRUE ("Writing")
      }
      frame "Restart" {
        n127 = Build Array(cluster{dbl[], dbl[]} {[], []} ("element"), w420, w416) -> (w419:cluster{dbl[], T2[]}[])
      }
    }
    "?" <- w54
    "XY Graph" <- w42
    n128 = node-c288() -> ()  [unwired: 1 in, 1 out]
  }
  n129 = timed-loop {
    shift-right: [w435] -> w30
    shift-left: w31 -> [w438]
    shift-right: [w440] -> w35
    shift-left: w33 -> [w441]
    shift-right: [w439] -> w34
    shift-left: w32 -> [w434]
    timing: w23 -> [_]
    timing-out: [_] -> w22
    tunnel: [w429] -> w6
    stop <- "Stop" stop-if-true
    n130 = node-c288() -> ()  [unwired: 1 in, 1 out]
    n131 = VISA Read(VISA resource name=w438, byte count=u32 2000, error in (no error)=w434) -> (VISA resource name out=w435:refnum<visa-resource-name>, read buffer=w431:string, return count=w436:u32, error out=w433:errorcluster)
    n132 = call <extravilib>:"Write.vi"("element"="Stop") -> ("channel"=w429:T17)  [unwired: 1 out]
    n133 = Greater Than 0?(x=w436) -> (x > 0?=w437:bool)
    n134 = case shown="True" w437 {
      tunnel: w441 -> [w445 w450]
      tunnel: [w445 w449] -> w440
      tunnel: w433 -> [w444 w448]
      tunnel: [w444 w447] -> w439
      tunnel: w431 -> [_ w446]
      frame False {
      }
      frame True {
        n135 = Enqueue Element(queue=w450, element=w446, error in (no error)=w448) -> (queue out=w449:refnum<queue>, error out=w447:errorcluster)  [unwired: 1 in, 1 out]
      }
    }
    n136 = node-c288() -> ()  [unwired: 1 in, 1 out]
  }
  n137 = while {
    tunnel: w17 -> [w456]
    tunnel: w16 -> [w453]
    shift-right: [w457] -> _
    shift-left: For_fsr_type_def."Waiting Room" -> [w458]
    shift-right: [w455] -> _
    shift-left: _ -> [w454]
    tunnel: w6 -> [w452]
    stop <- w451 stop-if-true
    n138 = case shown="\"Waiting Room\"" w458 {
      tunnel: [For_fsr_type_def."Waiting Room" For_fsr_type_def."Close File" For_fsr_type_def."Waiting Room" w489] -> w457
      tunnel: w456 -> [w470 w481 _ _]
      tunnel: w453 -> [w469 w480 _ _]
      tunnel: [w460 w472 w483 w488] -> w455
      tunnel: w454 -> [_ w477 w483 w488]
      frame "Create/Replace File", Default {
        n139 = Dequeue Element(queue=w470, error in (no error)=w469) -> (element=w467:string)  [unwired: 1 in, 3 out]
        n140 = Match Pattern(string=w467, regular expression="#") -> (before substring=w465:string, after substring=w464:string)  [unwired: 1 in, 2 out]
        n141 = call "subFILEmainGLD.vi"("String containing Filename"=w464, "String of Folder Names"=w465, "File Folder"="File Path") -> ("error out"=w461:errorcluster, "refnum out"=w462:refnum<file>)  [unwired: 7 in]
        n142 = Bundle("refnum out"=w462, "error out"=w461) -> (w460:T18)  [unwired: 1 in]
        n143 = local write "Creating"(FALSE ("Creating")) -> ()
      }
      frame "Write Data" {
        n144 = Unbundle By Name(w477) -> ("refnum out"=w476:refnum<file>, "error out"=w475:errorcluster)
        n145 = Dequeue Element(queue=w481, error in (no error)=w480) -> (element=w479:string)  [unwired: 1 in, 3 out]
        n146 = Write to Text File(file (use dialog)=w476, text=w479, error in=w475) -> (refnum out=w474:refnum<file>, error out=w473:errorcluster)  [unwired: 1 in, 1 out]
        n147 = Bundle("refnum out"=w474, "error out"=w473) -> (w472:T18)  [unwired: 1 in]
        n148 = local write "Writing"(FALSE ("Writing")) -> ()
      }
      frame "Close File" {
        n149 = Unbundle By Name(w483) -> ("refnum out"=w485:refnum<file>, "error out"=w484:errorcluster)
        n150 = Close File(refnum=w485, error in=w484) -> (error out=w486:errorcluster)  [unwired: 1 out]
        n151 = call <vilib>:"General Error Handler.vi"("error in (no error)"=w486) -> ()  [unwired: 10 in, 5 out]
      }
      frame "Waiting Room" {
        n152 = local read "Writing"() -> (w487:bool)
        n153 = case shown="False" w487 {
          tunnel: [w491 For_fsr_type_def."Write Data"] -> w489
          frame False {
            n154 = local read "Creating"() -> (w490:bool)
            n155 = case shown="True" w490 {
              tunnel: [For_fsr_type_def."Waiting Room" For_fsr_type_def."Create/Replace File"] -> w491
              frame False {
              }
              frame True {
              }
            }
          }
          frame True {
          }
        }
      }
    }
    n156 = call <extravilib>:"Read.vi"("channel"=w452) -> ("element"=w451:bool)  [unwired: 1 in, 1 out]
  }
  n157 = node-c288(w22) -> ()  [unwired: 1 out]
  n158 = Release Queue(queue=w35, error in (no error)=w34) -> (error out=w28:errorcluster)  [unwired: 1 in, 2 out]
  n159 = VISA Close(VISA resource name=w30, error in (no error)=w28) -> (error out=w29:errorcluster)
  n160 = call <vilib>:"Simple Error Handler.vi"("error in (no error)"=w29) -> ()  [unwired: 1 in, 8 out]
  n161 = node-c288() -> (w9:T11)  [unwired: 4 in]
  n162 = timed-loop {
    timing: w9 -> [_]
    timing-out: [_] -> w8
    tunnel: w6 -> [w496]
    stop <- w497 stop-if-true
    n163 = node-c288() -> ()  [unwired: 1 in, 1 out]
    n164 = local read "In Range?"() -> (w495:bool)
    n165 = call <extravilib>:"Read.vi"("channel"=w496) -> ("element"=w497:bool)  [unwired: 1 in, 1 out]
    n166 = case shown="True" w495 {
      frame False {
      }
      frame True {
        n167 = call <vilib>:"Beep.vi"("use system alert? (T)"=FALSE, "duration (msec)"=u32 1000, "frequency (Hz)"=u32 2500) -> ()  [unwired: 9 in]
      }
    }
    n168 = node-c288() -> ()  [unwired: 1 in, 1 out]
  }
  n169 = node-c288(w8) -> ()  [unwired: 1 out]
  n170 = node-c288(w20) -> ()  [unwired: 1 out]
  n171 = Release Queue(queue=w15, error in (no error)=w2) -> (error out=w14:errorcluster)  [unwired: 1 in, 2 out]
  n172 = call <vilib>:"Simple Error Handler.vi"("error in (no error)"=w14) -> ()  [unwired: 1 in, 8 out]
